vi "Msg.Event.Create.vi"(8 "Error (in)":errorcluster, 11 "Msg.Refs":T1) -> (0 "Error (out)":errorcluster, 3 "Msg.Refs (out)":T1)   [LabVIEW 2023, in "MessagingModule.lvlib"]
doc: "Used to create a user event."
uses:
  MessagingModule.lvlib
  Msg.Data.ctl
  Msg.Event.Ref.ctl
  Msg.Event.RegRef.ctl
  Msg.Q.Ref.ctl
  Msg.Noti.Ref.ctl
  Msg.Refs.ctl
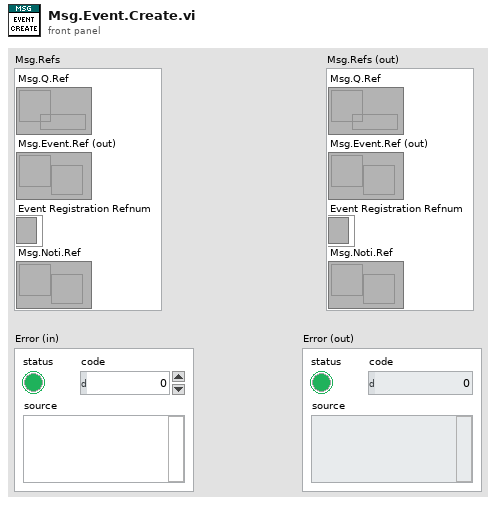
[diagram p1: front panel]
types:
  T1 = typedef "MessagingModule.lvlib/Msg.Refs.ctl" = cluster{"Msg.Q.Ref":T2, "Msg.Event.Ref (out)":T3, "Event Registration Refnum":T4, "Msg.Noti.Ref":T5}
  T2 = typedef "MessagingModule.lvlib/Msg.Q.Ref.ctl" = refnum<queue>
  T3 = typedef "MessagingModule.lvlib/Msg.Event.Ref.ctl" = refnum<user-event>
  T4 = typedef "MessagingModule.lvlib/Msg.Event.RegRef.ctl" = refnum<event-registration>
  T5 = typedef "MessagingModule.lvlib/Msg.Noti.Ref.ctl" = refnum<notifier>
  T6 = typedef "MessagingModule.lvlib/Msg.Data.ctl" = cluster{"Message":string, "Data":variant}
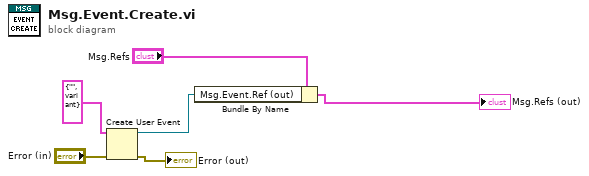
[diagram p0: block diagram]
diagram:
  n1 = Create User Event(user event datatype=T6 {"Message"="", "Data"=variant} ("Msg.Q.Data"), error in="Error (in)") -> (user event=w2:refnum<user-event>, error out=→"Error (out)":errorcluster)
  n2 = Bundle By Name(cluster="Msg.Refs", "Msg.Event.Ref (out)"=w2) -> (→"Msg.Refs (out)":T1)
